vi "Querry.vi"(8 "error in (no error)":errorcluster, 10 "PDU_req":T1={"Function Code"=1, "Data"=[], "RTU_DataBytes"=0}, 11 "MB_Master_TCP in":refnum<class "MB_Master_TCP.lvclass">) -> (0 "error out":errorcluster, 2 "PDU_resp":T1={"Function Code"=1, "Data"=[], "RTU_DataBytes"=0}, 3 "MB_Master_TCP out":refnum<class "MB_Master_TCP.lvclass">)   [LabVIEW 2012, in "MB Master.lvlib" / "MB_Master_TCP.lvclass"]
doc: "Transmits the PDU request and receives the PDU response as an atomic operation. The session is reserved by a mutex and the socket is already reserved."
uses:
  MB_Master_TCP.lvclass
  MB_PDU/MB_PDU_Cluster.ctl
  MB_Master_TCP.lvclass/MB_Master_TCP.ctl
  MB Master.lvlib
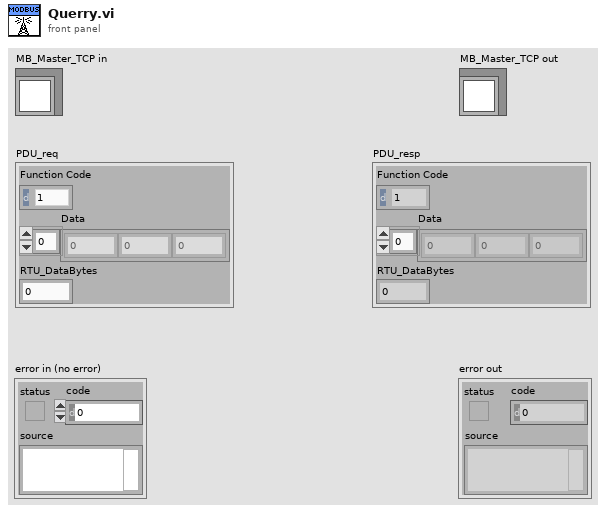
[diagram p1: front panel]
types:
  T1 = typedef "MB Master.lvlib/MB_PDU_Cluster.ctl" = cluster{"Function Code":u8, "Data":u8[], "RTU_DataBytes":i32}
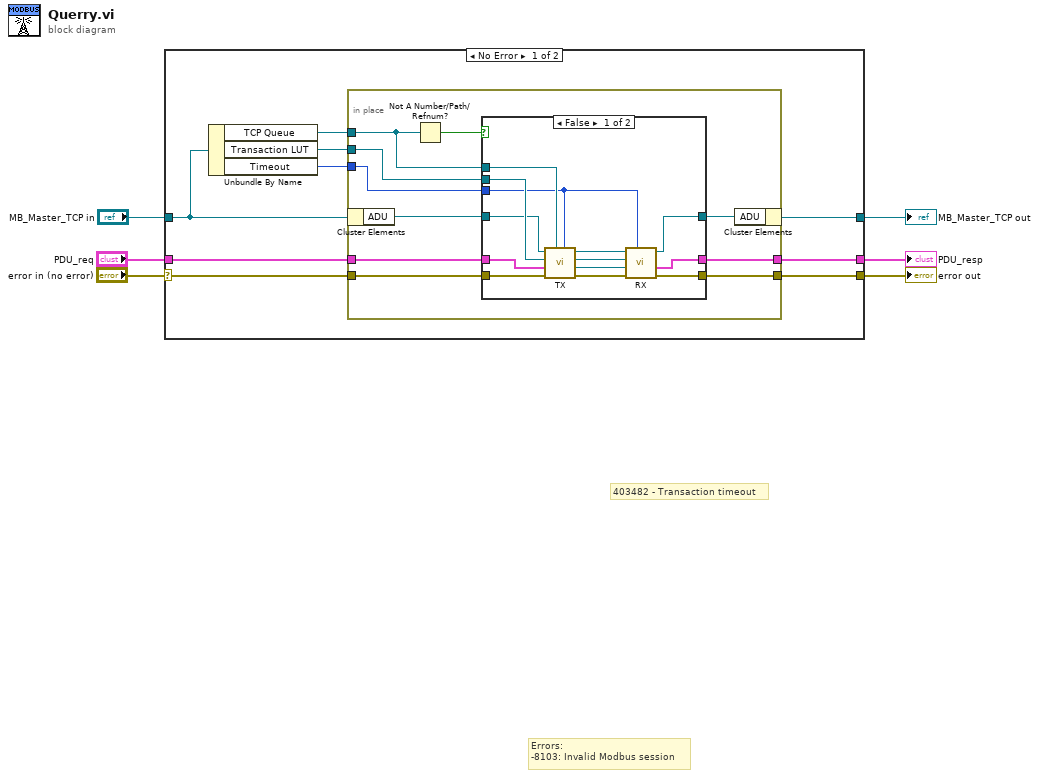
[diagram p0: block diagram]
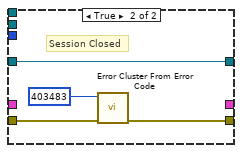
[diagram p2: hidden frame]
diagram:
  # "403482 - Transaction timeout"
  # "Errors:\n-8103: Invalid Modbus session"
  n1 = case shown="No Error" "error in (no error)" {
    selector: "error in (no error)" -> [w15 w44]
    tunnel: [w14 w44] -> w3
    tunnel: [w13 w43] -> w1
    tunnel: "MB_Master_TCP in" -> [w10 w43]
    tunnel: "PDU_req" -> [w12 _]
    tunnel: [w11 _] -> w2
    frame No Error {
      n2 = Unbundle By Name(w10) -> ("TCP Queue"=w9:refnum<queue>, "Transaction LUT"=w8:refnum<data-value>, "Timeout"=w7:i32)
      n3 = in-place {
        in-place-border: w15 -> [w24]
        in-place-border: [w25] -> w14
        in-place-border: w12 -> [w22]
        in-place-border: [w20] -> w11
        in-place-border: w9 -> [w17]
        in-place-border: w8 -> [w19]
        in-place-border: w7 -> [w18]
        n4 = in-place-cluster #1(w10) -> ("ADU"=w23:refnum<class "MB_ADU_TCP.lvclass">)
        n5 = Not A Number/Path/Refnum?(number/path/refnum=w17) -> (NaN/Path/Refnum?=w16:bool)
        n6 = case shown="False" w16 {
          tunnel: w24 -> [w38 w40]
          tunnel: w23 -> [w35 w42]
          tunnel: [w32 w42] -> w21
          tunnel: [w30 w39] -> w25
          tunnel: w22 -> [w34 _]
          tunnel: [w31 _] -> w20
          tunnel: w17 -> [w37 _]
          tunnel: w19 -> [w36 _]
          tunnel: w18 -> [w26 _]
          frame False {
            n7 = call "TX.vi"("timeout in ms (-1)"=w26, "TCP Queue"=w37, "error in (no error)"=w38, "PDU_req"=w34, "Transaction LUT in"=w36, "ADU in"=w35) -> ("error out"=w27:errorcluster, "Transaction Notifier"=w28:refnum<notifier>, "Transaction LUT out"=w29:refnum<data-value>, "ADU out"=w33:refnum<class "MB_ADU_TCP.lvclass">)  [unwired: 2 in]
            n8 = call "RX.vi"("Timeout (10000)"=w26, "error in (no error)"=w27, "Transaction Notifier"=w28, "Transaction LUT in"=w29, "ADU in"=w33) -> ("error out"=w30:errorcluster, "PDU_resp"=w31:T1, "ADU out"=w32:refnum<class "MB_ADU_TCP.lvclass">)  [unwired: 3 in, 1 out]
          }
          frame True {
            # "Session Closed"
            n9 = call <vilib>:"Error Cluster From Error Code.vi"("error in (no error)"=w40, "error code (0)"=403483) -> ("error out"=w39:errorcluster)  [unwired: 7 in]
          }
        }
        n10 = in-place-cluster #1("ADU"=w21) -> (w13:refnum<class "MB_Master_TCP.lvclass">)
      }
    }
    frame Error {
    }
  }
  "error out" <- w3
  "MB_Master_TCP out" <- w1
  "PDU_resp" <- w2
